vi "Link Custom Types.vi"(8 "error in (no error)":errorcluster, 11 "LV-Protoc in":refnum<class "LV-Protoc.lvclass">) -> (0 "error out":errorcluster, 3 "LV-Protoc out":refnum<class "LV-Protoc.lvclass">)   [LabVIEW 2020, in "LV-Protoc.lvlib" / "LV-Protoc.lvclass"]
uses:
  LV-Protoc.lvclass
  LV-Protoc.lvclass/LV-Protoc.ctl
  LV-Proto/Proto Type.ctl
  LV-Proto/LV-Proto.lvlib
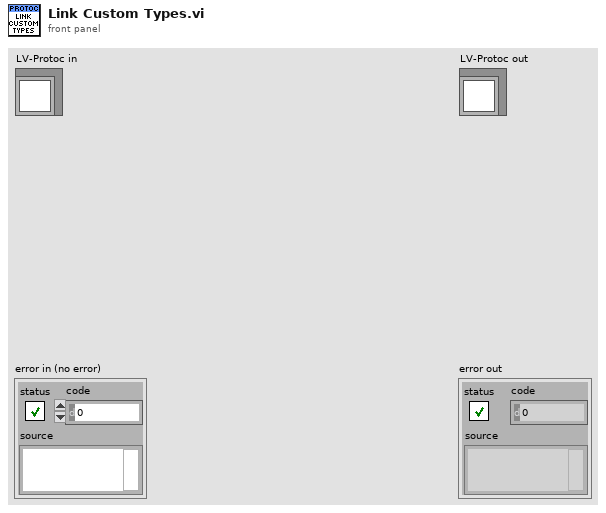
[diagram p1: front panel]
types:
  T1 = typedef "LV-Proto.lvlib/Proto Type.ctl" = enum16{"UNKNOWN", "double", "float", "int32", "int64", "uint32", "uint64", "sint32", "sint64", "fixed32", "fixed64", "sfixed32", "sfixed64", "bool", "string", "bytes", "enum", "map", "message"}
  T2 = typedef "LV-Proto.lvlib/Message.ctl" = cluster{"Name":string, "Fields":T3[], "Reserved Numbers":u32[], "Reserved Names":string[]}
  T3 = typedef "LV-Proto.lvlib/Field.ctl" = cluster{"Name":string, "Number":u32, "Optional":bool, "Repeated":bool, "Type":T4, "Key Type":T4, "Value Type":T4}
  T4 = typedef "LV-Proto.lvlib/Type.ctl" = cluster{"Type":T1, "Subtype":string}
  T5 = typedef "LV-Protoc.lvlib/Custom Type.ctl" = enum16{"enum", "message"}
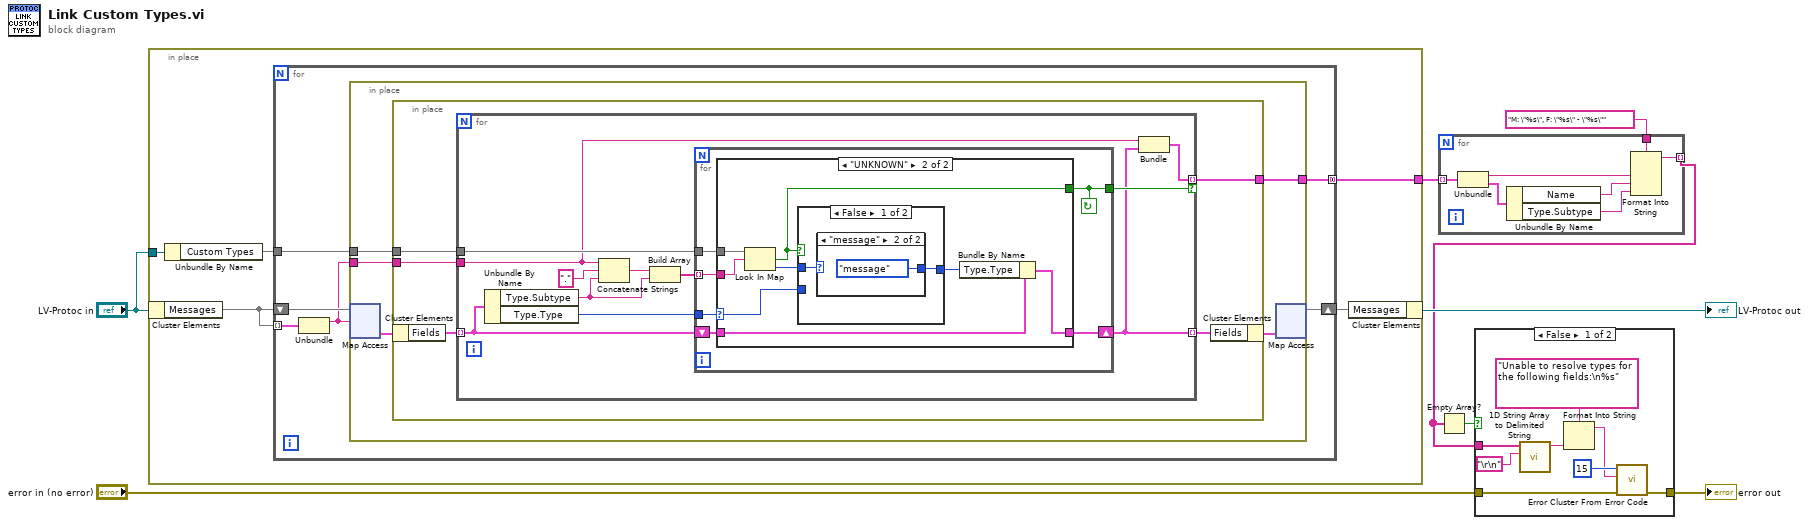
[diagram p0: block diagram]
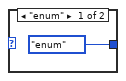
[diagram p4: hidden frame]
diagram:
  n1 = in-place {
    in-place-border: "LV-Protoc in" -> [w12]
    in-place-border: [w9] -> w6
    n2 = in-place-cluster #1("LV-Protoc in") -> ("Messages"=w13:map{string, T2})
    n3 = Unbundle By Name(w12) -> ("Custom Types"=w11:map{string, T5})
    n4 = for {
      tunnel: w13 -> [w18] mode=indexing
      shift-right: [w16] -> w10
      shift-left: w13 -> [w19]
      tunnel: w11 -> [w17]
      tunnel: [w14] -> w9 mode=concatenating
      n5 = Unbundle(w18) -> ("Name"=w15:string)  [unwired: 1 out]
      n6 = in-place {
        in-place-border: w17 -> [w23]
        in-place-border: w15 -> [w21]
        in-place-border: [w20] -> w14
        n7 = in-place-map #2(w19, w15) -> (w24:T2)  [unwired: 1 in, 1 out]
        n8 = in-place {
          in-place-border: w23 -> [w28]
          in-place-border: w21 -> [w26]
          in-place-border: [w25] -> w20
          n9 = in-place-cluster #3(w24) -> ("Fields"=w29:T3[])
          n10 = for {
            tunnel: w29 -> [w38] mode=indexing
            tunnel: w28 -> [w39]
            tunnel: [w31] -> w27 mode=indexing
            tunnel: w26 -> [w32]
            tunnel: [w30] -> w25 mode=indexing if=w33
            n11 = Unbundle By Name(w38) -> ("Type.Subtype"=w35:string, "Type.Type"=w40:T1)
            n12 = Concatenate Strings(w32, "." ("string"), w35) -> (w36:string)
            n13 = Build Array(w36, w35) -> (w34:string[])
            n14 = for {
              tunnel: w40 -> [w46]
              tunnel: w39 -> [w45]
              shift-right: [w44] -> w31
              shift-left: w38 -> [w43]
              tunnel: w34 -> [w42] mode=indexing
              tunnel: [w41] -> w33
              stop <- w41 continue-if-true
              n15 = case shown="\"UNKNOWN\"" w46 {
                selector: w46 -> [_ w52]
                tunnel: w45 -> [_ w55]
                tunnel: [w47 w50] -> w44
                tunnel: w43 -> [w47 w54]
                tunnel: w42 -> [_ w49]
                tunnel: [_ w48] -> w41
                frame Default {
                }
                frame "UNKNOWN" {
                  n16 = Look In Map(map=w55, key=w49) -> (key not found?=w48:bool, value=w53:T5)  [unwired: 1 in]
                  n17 = case shown="False" w48 {
                    tunnel: w53 -> [w57 _]
                    tunnel: w52 -> [_ w60]
                    tunnel: [w56 w60] -> w51
                    frame False {
                      n18 = case shown="\"message\"" w57 {
                        tunnel: [Proto_Type."enum" ("Type") Proto_Type."message" ("Type")] -> w56
                        frame "enum" {
                        }
                        frame "message" {
                        }
                      }
                    }
                    frame True {
                    }
                  }
                  n19 = Bundle By Name(cluster=w54, "Type.Type"=w51) -> (w50:T3)
                }
              }
            }
            n20 = Bundle("Name"=w32, "Field"=w31) -> (w30:cluster{"Name":string, "Field":T3})  [unwired: 1 in]
          }
          n21 = in-place-cluster #3("Fields"=w27) -> (w22:T2)
        }
        n22 = in-place-map #2(w22) -> (w16:map{string, T2})  [unwired: 1 in, 2 out]
      }
    }
    n23 = in-place-cluster #1("Messages"=w10) -> (→"LV-Protoc out":refnum<class "LV-Protoc.lvclass">)
  }
  n24 = for {
    tunnel: w6 -> [w67] mode=indexing
    tunnel: "M: \"%s\", F: \"%s\" - \"%s\"" -> [w65]
    tunnel: [w61] -> w3 mode=indexing
    n25 = Unbundle(w67) -> ("Name"=w64:string, "Field"=w66:T3)
    n26 = Unbundle By Name(w66) -> ("Name"=w63:string, "Type.Subtype"=w62:string)
    n27 = Format Into String(format string=w65, w64, w63, w62) -> (resulting string=w61:string)  [unwired: 2 in, 1 out]
  }
  n28 = Empty Array?(array=w3) -> (empty?=w4:bool)
  n29 = case shown="False" w4 {
    tunnel: w3 -> [w75 _]
    tunnel: [w69 w76] -> w2
    tunnel: "error in (no error)" -> [w68 w76]
    frame False {
      n30 = call <vilib>:"1D String Array to Delimited String.vi"("delimiter"="\r\n", "string array"=w75) -> ("delimited string"=w72:string)  [unwired: 9 in]
      n31 = Format Into String(format string="Unable to resolve types for the following fields:\n%s", w72) -> (resulting string=w70:string)  [unwired: 2 in, 1 out]
      n32 = call <vilib>:"Error Cluster From Error Code.vi"("error in (no error)"=w68, "error message (\"\")"=w70, "error code (0)"=15) -> ("error out"=w69:errorcluster)  [unwired: 6 in]
    }
    frame True {
    }
  }
  "error out" <- w2
